vi "习7.2.vi"() -> ()   [LabVIEW 2017]
panel:
  out "波形图":cluster{dbl[]}[](graph)
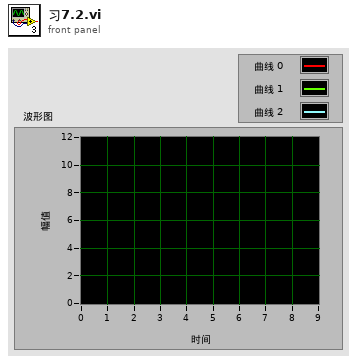
[diagram p1: front panel]
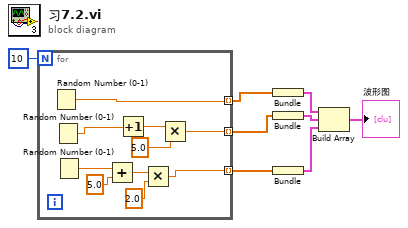
[diagram p0: block diagram]
diagram:
  n1 = for {
    N: 10 -> [_]
    tunnel: [w15] -> w8 mode=indexing
    tunnel: [w16] -> w4 mode=indexing
    tunnel: [w11] -> w3 mode=indexing
    n2 = Random Number (0-1)() -> (number: 0 to 1=w15:dbl)
    n3 = Random Number (0-1)() -> (number: 0 to 1=w9:dbl)
    n4 = Random Number (0-1)() -> (number: 0 to 1=w10:dbl)
    n5 = Add(x=w10, y=5.0) -> (x+y=w13:dbl)
    n6 = Increment(x=w9) -> (x+1=w18:dbl)
    n7 = Multiply(x=w13, y=2.0) -> (x*y=w11:dbl)
    n8 = Multiply(x=w18, y=5.0) -> (x*y=w16:dbl)
  }
  n9 = Bundle(w8) -> (w7:cluster{dbl[]})  [unwired: 1 in]
  n10 = Bundle(w4) -> (w2:cluster{dbl[]})  [unwired: 1 in]
  n11 = Bundle(w3) -> (w1:cluster{dbl[]})  [unwired: 1 in]
  n12 = Build Array(w7, w2, w1) -> (→"波形图":cluster{dbl[]}[])
